vi "Save Printer Settings.vi"(8 "Error in":errorcluster caption="Error in (no error)", 10 "Printer Settings":T1={"Project"={"Paths"=FALSE, "Descriptions"=FALSE, "Memory"=FALSE, "Options"=TRUE, "Symbols"=TRUE}, "VI Member"={"Memory"=TRUE, "By Folder"=TRUE, "By Tree"=TRUE, "By List"=TRUE, "Methods"=TRUE, "Method Options"={"Front Panels"=TRUE, "Options"=TRUE, "Controls"=TRUE}, "List Detail Level"=enum."None", "Methods Detail Level"=enum."None", "Controls Detail Level"=enum."None"}, "Interface"={"Memory"=TRUE, "By List"=TRUE, "Details"=TRUE, "Detail Options"={"Description"=TRUE, "Properties"=TRUE, "Inheritance"=TRUE, "Inheritance Options"={"Parent Interfaces"=TRUE, "Friends"=TRUE}}, "List Detail Level"=enum."None", "Controls Detail Level"=enum."None", "Methods Detail Level"=enum."None", "Controls Scope"={"Public"=TRUE, "Protected"=TRUE, "Community"=TRUE, "Private"=TRUE, "Unknown"=TRUE}, "Methods Scope"={"Public"=TRUE, "Protected"=TRUE, "Community"=TRUE, "Private"=TRUE, "Unknown"=TRUE}}, "Class"={"Memory"=TRUE, "By Folder"=TRUE, "By Tree"=TRUE, "By List"=TRUE, "Details"=TRUE, "Detail Options"={"Description"=TRUE, "Properties"=TRUE, "Inheritance"=TRUE, "Inheritance Options"={"Parent Classes"=TRUE, "Parent Interfaces"=TRUE, "Parent Libraries"=TRUE, "Friends"=TRUE}}, "CPD Detail Level"=enum."None", "List Detail Level"=enum."None", "Controls Detail Level"=enum."None", "Methods Detail Level"=enum."None", "Set Accessor Detail Level"=enum."None", "Get Accessor Detail Level"=enum."None", "Controls Scope"={"Public"=TRUE, "Protected"=TRUE, "Community"=TRUE, "Private"=TRUE, "Unknown"=TRUE}, "Methods Scope"={"Public"=TRUE, "Protected"=TRUE, "Community"=TRUE, "Private"=TRUE, "Unknown"=TRUE}, "Get Accessors Scope"={"Public"=TRUE, "Protected"=TRUE, "Community"=TRUE, "Private"=TRUE, "Unknown"=TRUE}, "Set Accessors Scope"={"Public"=TRUE, "Protected"=TRUE, "Community"=TRUE, "Private"=TRUE, "Unknown"=TRUE}}, "Library"={"Memory"=TRUE, "By Folder"=TRUE, "By Tree"=TRUE, "By List"=TRUE, "Details"=TRUE, "Detail Options"={"Description"=TRUE, "Properties"=TRUE, "Friends"=TRUE, "Child Libraries"=TRUE}, "List Detail Level"=enum."None", "Methods Detail Level"=enum."None", "Controls Detail Level"=enum."None", "Methods Scope"={"Public"=TRUE, "Protected"=TRUE, "Community"=TRUE, "Private"=TRUE, "Unknown"=TRUE}, "Controls Scope"={"Public"=TRUE, "Protected"=TRUE, "Community"=TRUE, "Private"=TRUE, "Unknown"=TRUE}}, "Control Member"={"Memory"=TRUE, "By Folder"=TRUE, "By Tree"=TRUE, "By List"=TRUE, "Controls"=TRUE, "List Detail Level"=enum."None", "Controls Detail Level"=enum."None"}, "Format Options"={"Background"={"Public Scope"={"Option"=FALSE, "Color"=0, "Operator"=FALSE}, "Protected Scope"={"Option"=FALSE, "Color"=0, "Operator"=FALSE}, "Community Scope"={"Option"=FALSE, "Color"=0, "Operator"=FALSE}, "Private Scope"={"Option"=FALSE, "Color"=0, "Operator"=FALSE}, "Unknown Scope"={"Option"=FALSE, "Color"=0, "Operator"=FALSE}, "Auto Error Handling"={"Option"=FALSE, "Color"=0, "Operator"=FALSE}, "Inline"={"Option"=FALSE, "Color"=0, "Operator"=FALSE}, "Separate CC"={"Option"=FALSE, "Color"=0, "Operator"=FALSE}, "Execution Priority Normal"={"Option"=FALSE, "Color"=0, "Operator"=FALSE}, "Reentrancy Non-RE"={"Option"=FALSE, "Color"=0, "Operator"=FALSE}}, "Bookmark Options"={"Bookmarks as New Line in VI Descriptions"=TRUE, "Unique Bookmark Tags Only"=TRUE, "Include Tag and Text"=TRUE}}, "Library Scope"={"Public"=TRUE, "Community"=TRUE, "Private"=TRUE, "Unknown"=TRUE}, "LLB"={"Methods"=TRUE, "Controls"=TRUE, "Methods Detail Level"=enum."None", "Controls Detail Level"=enum."None"}, "Bookmark Settings Map"={}} caption="Doc Options", 11 "Settings Path":path) -> (0 "Error out":errorcluster)   [LabVIEW 2023, in "VIDoc Printer.lvlib" / "Printer Settings.lvclass"]
uses:
  Printer Settings.lvclass
  Printer Settings Cluster.ctl
  Project Settings.ctl
  VI Settings.ctl
  Detail Level Enum.ctl
  Interface Settings.ctl
  Scope Settings.ctl
  Class Settings.ctl
  Library Settings.ctl
  Control Settings.ctl
  Formatting Options.ctl
  Background Formatting Cluster.ctl
  Bookmark Options.ctl
  LLB Settings.ctl
  e450ed71-4968-4477-8672-58ac8a0708d9.vi
  <vilib>/JDP Science/JSONtext/Variant to JSON Text.vi
  <vilib>/JDP Science/JSONtext/LVClass Serializer/JSONtext LVClass Serializer.lvclass
  Printer Settings.lvclass/Printer Settings.ctl
  VIDoc Settings/VIDoc Settings.lvclass
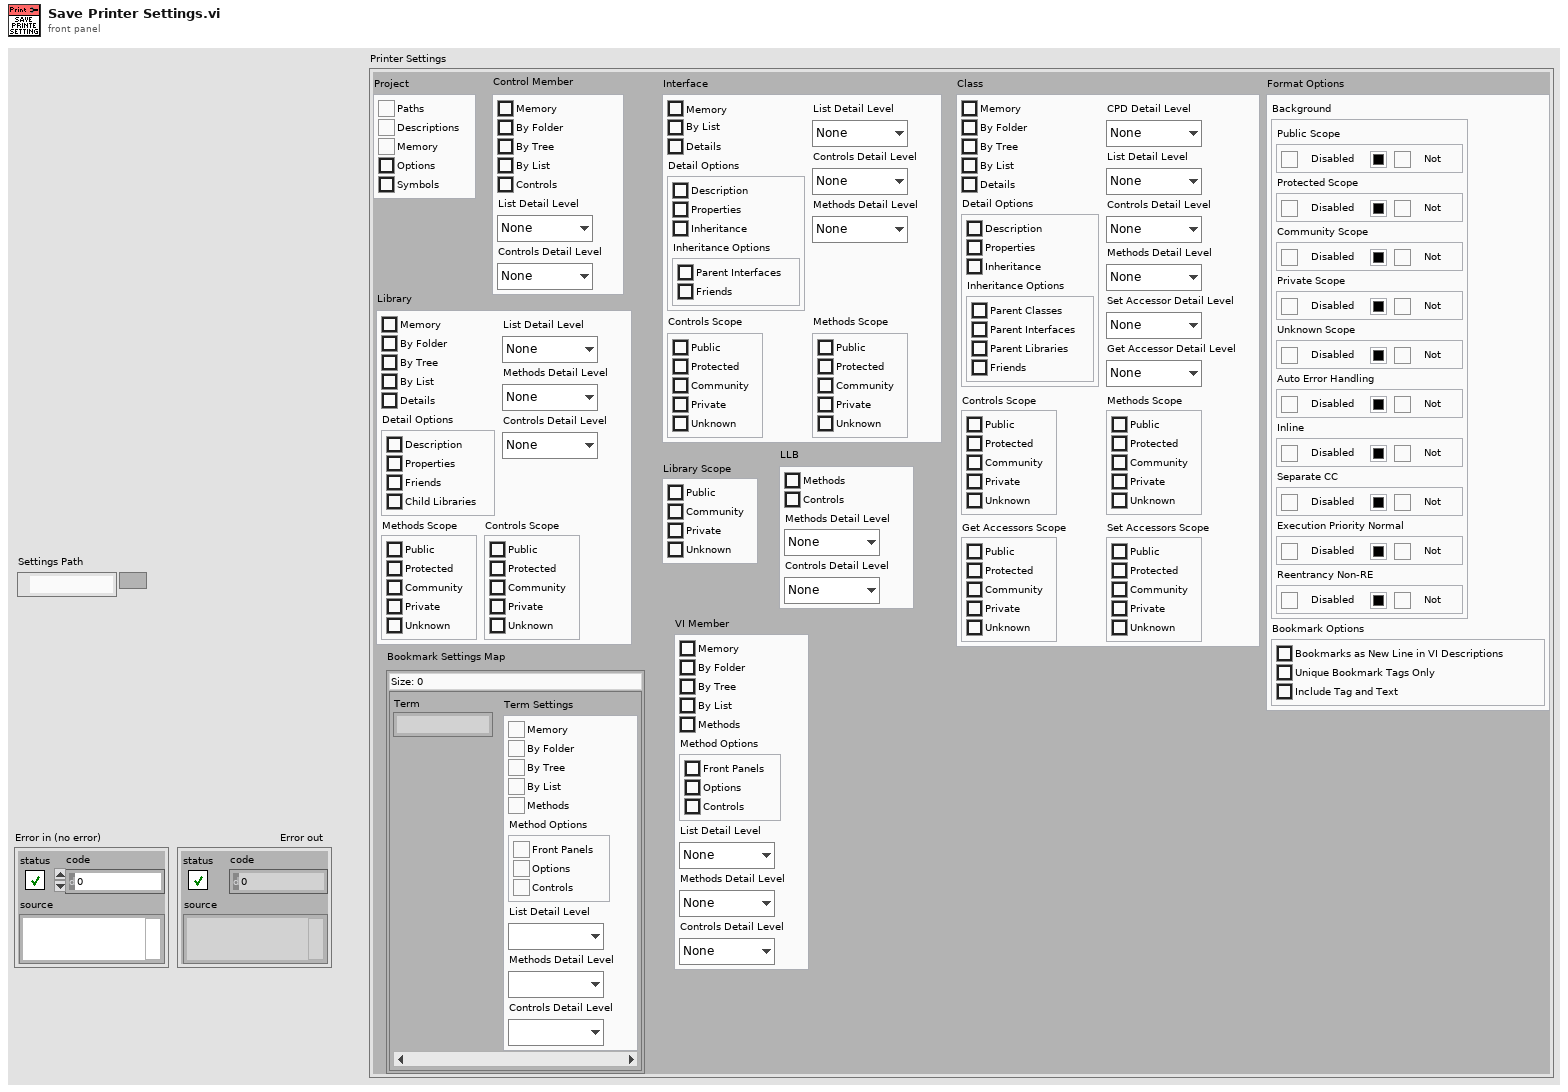
[diagram p1: front panel]
types:
  T1 = typedef "VIDoc Printer.lvlib/Printer Settings.lvclass/Printer Settings Cluster.ctl" = cluster{"Project":T2, "VI Member":T3, "Interface":T5, "Class":T7, "Library":T8, "Control Member":T9, "Format Options":T10, "Library Scope":cluster{"Public":bool, "Community":bool, "Private":bool, "Unknown":bool}, "LLB":T13, "Bookmark Settings Map":map{string, T3}}
  T2 = typedef "VIDoc Printer.lvlib/Printer Settings.lvclass/Project Settings.ctl" = cluster{"Paths":bool, "Descriptions":bool, "Memory":bool, "Options":bool, "Symbols":bool}
  T3 = typedef "VIDoc Printer.lvlib/Printer Settings.lvclass/VI Settings.ctl" = cluster{"Memory":bool, "By Folder":bool, "By Tree":bool, "By List":bool, "Methods":bool, "Method Options":cluster{"Front Panels":bool, "Options":bool, "Controls":bool}, "List Detail Level":T4, "Methods Detail Level":T4, "Controls Detail Level":T4}
  T4 = typedef "VIDoc Printer.lvlib/Printer Settings.lvclass/Detail Level Enum.ctl" = enum16{"None", "Minimal", "Standard", "Full"}
  T5 = typedef "VIDoc Printer.lvlib/Printer Settings.lvclass/Interface Settings.ctl" = cluster{"Memory":bool, "By List":bool, "Details":bool, "Detail Options":cluster{"Description":bool, "Properties":bool, "Inheritance":bool, "Inheritance Options":cluster{"Parent Interfaces":bool, "Friends":bool}}, "List Detail Level":T4, "Controls Detail Level":T4, "Methods Detail Level":T4, "Controls Scope":T6, "Methods Scope":T6}
  T6 = typedef "VIDoc Printer.lvlib/Printer Settings.lvclass/Scope Settings.ctl" = cluster{"Public":bool, "Protected":bool, "Community":bool, "Private":bool, "Unknown":bool}
  T7 = typedef "VIDoc Printer.lvlib/Printer Settings.lvclass/Class Settings.ctl" = cluster{"Memory":bool, "By Folder":bool, "By Tree":bool, "By List":bool, "Details":bool, "Detail Options":cluster{"Description":bool, "Properties":bool, "Inheritance":bool, "Inheritance Options":cluster{"Parent Classes":bool, "Parent Interfaces":bool, "Parent Libraries":bool, "Friends":bool}}, "CPD Detail Level":T4, "List Detail Level":T4, "Controls Detail Level":T4, "Methods Detail Level":T4, "Set Accessor Detail Level":T4, "Get Accessor Detail Level":T4, "Controls Scope":T6, "Methods Scope":T6, "Get Accessors Scope":T6, "Set Accessors Scope":T6}
  T8 = typedef "VIDoc Printer.lvlib/Printer Settings.lvclass/Library Settings.ctl" = cluster{"Memory":bool, "By Folder":bool, "By Tree":bool, "By List":bool, "Details":bool, "Detail Options":cluster{"Description":bool, "Properties":bool, "Friends":bool, "Child Libraries":bool}, "List Detail Level":T4, "Methods Detail Level":T4, "Controls Detail Level":T4, "Methods Scope":T6, "Controls Scope":T6}
  T9 = typedef "VIDoc Printer.lvlib/Printer Settings.lvclass/Control Settings.ctl" = cluster{"Memory":bool, "By Folder":bool, "By Tree":bool, "By List":bool, "Controls":bool, "List Detail Level":T4, "Controls Detail Level":T4}
  T10 = typedef "VIDoc Printer.lvlib/Printer Settings.lvclass/Formatting Options.ctl" = cluster{"Background":cluster{"Public Scope":T11, "Protected Scope":T11, "Community Scope":T11, "Private Scope":T11, "Unknown Scope":T11, "Auto Error Handling":T11, "Inline":T11, "Separate CC":T11, "Execution Priority Normal":T11, "Reentrancy Non-RE":T11}, "Bookmark Options":T12}
  T11 = typedef "VIDoc Printer.lvlib/Printer Settings.lvclass/Background Formatting Cluster.ctl" = cluster{"Option":bool, "Color":u32, "Operator":bool}
  T12 = typedef "VIDoc Printer.lvlib/Printer Settings.lvclass/Bookmark Options.ctl" = cluster{"Bookmarks as New Line in VI Descriptions":bool, "Unique Bookmark Tags Only":bool, "Include Tag and Text":bool}
  T13 = typedef "VIDoc Printer.lvlib/Printer Settings.lvclass/LLB Settings.ctl" = cluster{"Methods":bool, "Controls":bool, "Methods Detail Level":T4, "Controls Detail Level":T4}
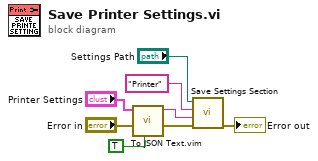
[diagram p0: block diagram]
diagram:
  n1 = call "To JSON Text.vim"("Pretty Print?"=TRUE, "error in (no error)"="Error in", "Anything"="Printer Settings") -> ("error out"=w6:errorcluster, "<JSON>"=w4:string)  [unwired: 7 in]
  n2 = call "Save Settings Section.vi"("Error in"=w6, "JSON Object"=w4, "Section Name"="Printer", "JSON Settings Path"="Settings Path") -> ("Error out"=→"Error out":errorcluster)  [unwired: 7 in]
